vi "Load Dynamic Dependency.vi"(7 "SMO in":refnum<class "SMO.lvclass">, 8 "error in (no error)":errorcluster, 10 "HAL Folder (Subsystems)":string="Subsystems", 11 "Class Name":string) -> (0 "error out":errorcluster, 3 "SMO out":refnum<class "SMO.lvclass">)   [LabVIEW 2017]
uses:
  <vilib>/JKI/JKI SMO/SMO/SMO.lvclass
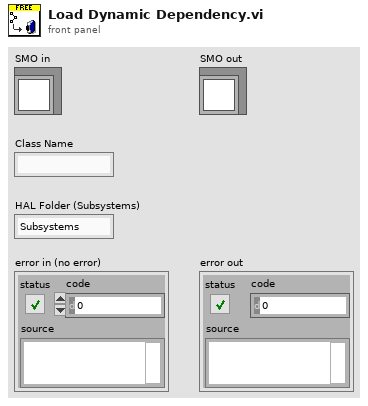
[diagram p1: front panel]
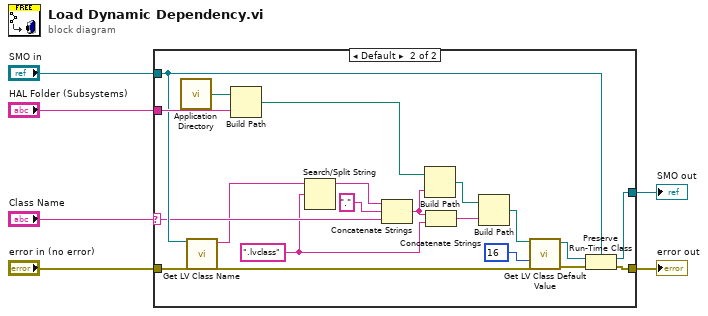
[diagram p0: block diagram]
diagram:
  n1 = case shown="Default" "Class Name" {
    selector: "Class Name" -> [_ w13]
    tunnel: "SMO in" -> [w8 w17]
    tunnel: "error in (no error)" -> [w7 w15]
    tunnel: [w7 w20] -> w3
    tunnel: [w8 w19] -> w5
    tunnel: "HAL Folder (Subsystems)" -> [_ w18]
    frame "" {
    }
    frame Default {
      w10 = ".lvclass" ("search string/char (-)")
      n2 = call <vilib>:"Application Directory.vi"() -> ("Application Directory"=w27:path)
      n3 = call <vilib>:"Get LV Class Name.vi"("error in (no error)"=w15, "object"=w17) -> ("error out"=w14:errorcluster, "class name"=w9:string)  [unwired: 8 in]
      n4 = Build Path(base path=w27, name or relative path=w18) -> (appended path=w26:path)
      n5 = Search/Split String(string=w9, search string/char (-)=w10) -> (substring before match=w16:string)  [unwired: 1 in, 2 out]
      n6 = Concatenate Strings(w16, "." ("string"), w13) -> (w11:string)
      n7 = Build Path(base path=w26, name or relative path=w11) -> (appended path=w23:path)
      n8 = Concatenate Strings(w11, w10) -> (w12:string)
      n9 = Build Path(base path=w23, name or relative path=w12) -> (appended path=w22:path)
      n10 = call <vilib>:"Get LV Class Default Value.vi"("error in (no error)"=w14, "options"=u32 16, "class path"=w22) -> ("error out"=w24:errorcluster, "object"=w25:refnum<class>)  [unwired: 7 in]
      n11 = Preserve Run-Time Class(object in=w25, error in=w24, 2:w17) -> (object out=w19:refnum<class "SMO.lvclass">, error out=w20:errorcluster)
    }
  }
  "SMO out" <- w5
  "error out" <- w3
